vi "event.vi"() -> ()   [LabVIEW 2020]
panel:
  out "String":string
  in  "stop":bool
  in  "B":bool
  in  "A":bool
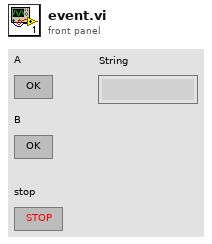
[diagram p1: front panel]
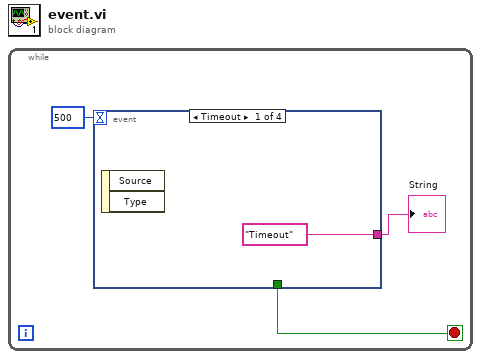
[diagram p0: block diagram]
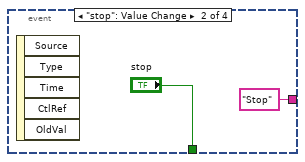
[diagram p2: hidden frame]
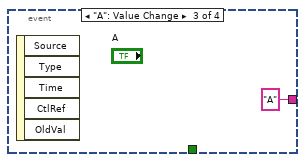
[diagram p3: hidden frame]
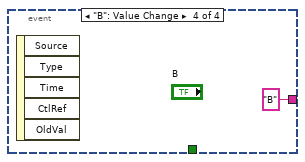
[diagram p4: hidden frame]
diagram:
  n1 = while {
    stop <- w2 stop-if-true
    n2 = event shown="[0] Timeout" {
      selector: _ -> [_ _ _ _]
      dyn-events: _ -> [_ _ _ _]
      timeout: 500 -> [_ _ _ _]
      tunnel: ["Timeout" "Stop" "A" "B"] -> w1
      tunnel: [_ "stop" _ _] -> w2
      event Timeout {
        n3 = event-data() -> ()  [unwired: 1 in, 2 out]
      }
      event "stop": Value Change {
        n4 = event-data() -> ()  [unwired: 1 in, 5 out]
      }
      event "A": Value Change {
        n5 = event-data() -> ()  [unwired: 1 in, 5 out]
      }
      event "B": Value Change {
        n6 = event-data() -> ()  [unwired: 1 in, 5 out]
      }
    }
    "String" <- w1
  }
